vi "DataGridView_Create.vi"(0 "reference in":refnum<class "DataGridView.lvclass">, 5 "DataGridView":refnum<k24>, 11 "error in (no error)":errorcluster) -> (4 "reference out":refnum<class "DataGridView.lvclass">, 15 "error out":errorcluster)   [LabVIEW 2018, in "DataGridView.lvclass"]
doc: "Creates the class\n\nHides the DataGridView for faster initialisation."
uses:
  DataGridView.lvclass
  System.Windows.Forms
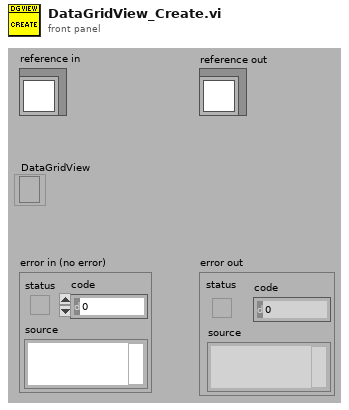
[diagram p1: front panel]
types:
  T1 = typedef "DataGridView.lvclass/ObjectAttributes.ctl" = cluster{"DataGridView":refnum<k24>, "SelectionChangedEvent":refnum<user-event>, "SelectionChanged callback ref":refnum<k27>, "LastSelectedRowIndex":i32, "CellClickEvent":refnum<user-event>, "CellClick callback refnum":refnum<k27>}
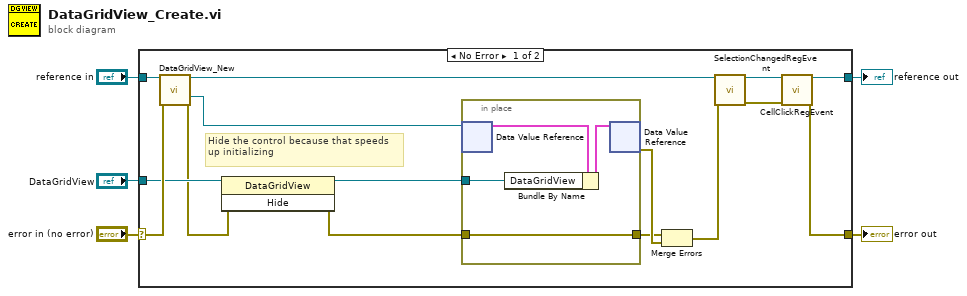
[diagram p0: block diagram]
diagram:
  n1 = case shown="No Error" "error in (no error)" {
    selector: "error in (no error)" -> [w19 w26]
    tunnel: [w8 w26] -> w4
    tunnel: "reference in" -> [w20 w25]
    tunnel: [w6 w25] -> w2
    tunnel: "DataGridView" -> [w14 _]
    frame No Error {
      # "Hide the control because that speeds up initializing"
      n2 = call "DataGridView_New.vi"("reference in"=w20, "error in (no error)"=w19) -> ("reference out"=w9:refnum<class "DataGridView.lvclass">, "DVRRefOut"=w17:refnum<data-value>, "error out"=w13:errorcluster)  [unwired: 10 in, 1 out]
      n3 = invoke class="DataGridView" method="Hide"(reference=w14, error in=w13) -> (reference out=w12:refnum<k24>, error out=w11:errorcluster)  [unwired: 1 in, 1 out]
      n4 = in-place {
        in-place-border: w11 -> [w22]
        in-place-border: [w22] -> w16
        in-place-border: w12 -> [w21]
        n5 = in-place-dvr #1(w17) -> (w23:T1)  [unwired: 1 out]
        n6 = Bundle By Name(cluster=w23, "DataGridView"=w21) -> (w24:T1)
        n7 = in-place-dvr #1(w24) -> (w18:errorcluster)  [unwired: 1 out]
      }
      n8 = Merge Errors(w16, w18) -> (w15:errorcluster)
      n9 = call "SelectionChangedRegEvent.vi"("reference in"=w9, "error in (no error)"=w15) -> ("reference out"=w7:refnum<class "DataGridView.lvclass">, "error out"=w10:errorcluster)  [unwired: 12 in]
      n10 = call "CellClickRegEvent.vi"("reference in"=w7, "error in (no error)"=w10) -> ("reference out"=w6:refnum<class "DataGridView.lvclass">, "error out"=w8:errorcluster)  [unwired: 12 in]
    }
    frame Error {
      # "VI-TechBaseTemplate_Simple_4x4x4"
    }
  }
  "error out" <- w4
  "reference out" <- w2
